vi "Q Vision_2016 Object Calcs.vi"(4 "Threshhold":i32=50, 6 "ColorMask Low/High":u8[][](array[numeric])=[[0, 100], [200, 255], [170, 230]], 7 "ColorSpace":T1, 8 "error in (no error)":errorcluster, 10 "Image in":T3) -> (0 "error out":errorcluster, 3 "Object Params out":T2 {"Deg_Up" format="%.2f"; "Deg_Rt" format="%.2f"; "Dist_ft" format="%.1f"})   [LabVIEW 2016]
uses:
  <vilib>/vision/Image Controls.llb/IMAQ Image.ctl
  Typedefs/typedef_cluster_Object Params.ctl
  Quick Vision/Typedefs/typedef_enum_ColorSpace.ctl
panel:
  out "B/W Image":i16[][](graph)
  out "Image Pixels (U32)":u32[][](array[numeric]) format="%08x"
  out "B/W Image_Object":i16[][](graph)
  # "R"
  # "G"
  # "B"
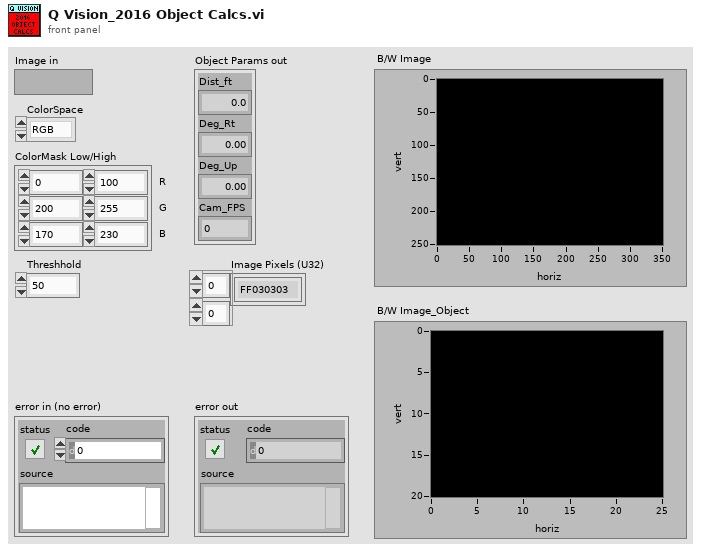
[diagram p1: front panel]
types:
  T1 = typedef "typedef_enum_ColorSpace.ctl" = enum16{"RGB", "HSL"}
  T2 = typedef "typedef_cluster_Object Params.ctl" = cluster{"Dist_ft":dbl, "Deg_Rt":dbl, "Deg_Up":dbl, "Cam_FPS":dbl}
  T3 = typedef "IMAQ Image.ctl" = refnum<image>
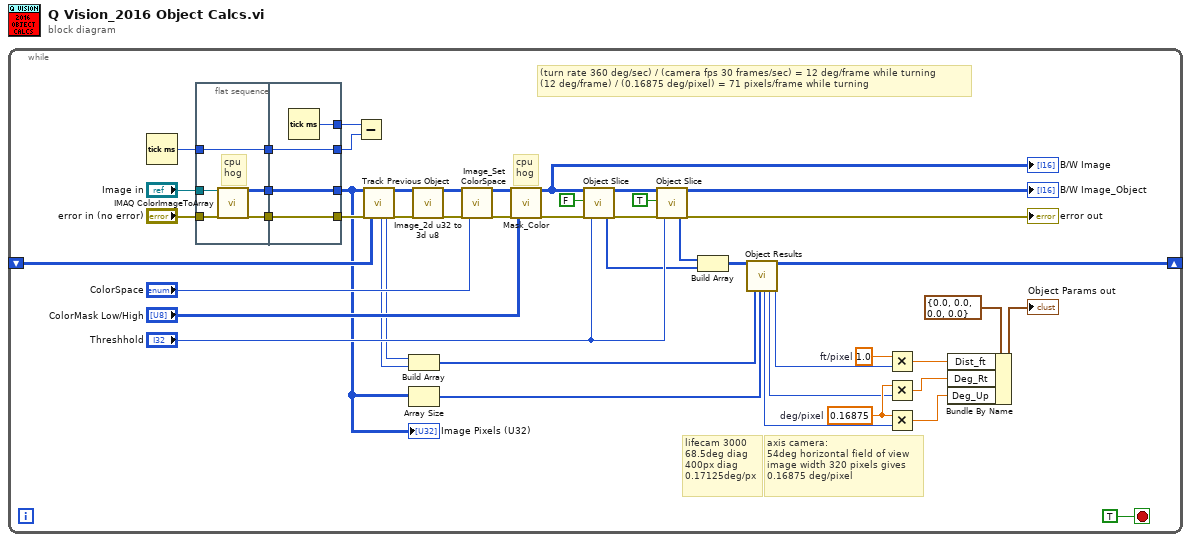
[diagram p0: block diagram]
diagram:
  n1 = while {
    shift-right: [w8] -> _
    shift-left: _ -> [w20]
    stop <- TRUE stop-if-true
    w7 = 1.0  # ft/pixel
    w28 = 0.16875  # deg/pixel
    # "lifecam 3000\n68.5deg diag\n400px diag\n0.17125deg/px"
    # "(turn rate 360 deg/sec) / (camera fps 30 frames/sec) = 12 deg/frame while turning\n(12 deg/frame) / (0.16875 deg/pixel) = 71 pixels/frame while turning"
    # "axis camera:\n54deg horizontal field of view\nimage width 320 pixels gives\n0.16875 deg/pixel"
    # "cpu\nhog"
    n2 = Tick Count (ms)() -> (millisecond timer value=w36:u32)
    n3 = flat-sequence {
      tunnel: [w52] -> w46
      tunnel: [w50] -> w45
      tunnel: [w51] -> w44
      tunnel: w36 -> [w50]
      tunnel: "Image in" -> [w49]
      tunnel: "error in (no error)" -> [w48]
      tunnel: [w54] -> w19
      tunnel: [w55] -> w30
      tunnel: [w56] -> w17
      tunnel: w46 -> [w56]
      tunnel: w45 -> [w55]
      tunnel: w44 -> [w54]
      tunnel: [w53] -> w31
      frame #0 {
        # "cpu\nhog"
        n4 = call "IMAQ ColorImageToArray"("Image"=w49, "error in (no error)"=w48) -> ("Image Pixels (U32)"=w52:u32[][], "error out"=w51:errorcluster)  [unwired: 2 in, 1 out]
      }
      frame #1 {
        n5 = Tick Count (ms)() -> (millisecond timer value=w53:u32)
      }
    }
    n6 = Subtract(x=w31, y=w30) -> ()  [unwired: 1 out]
    n7 = call "Track Previous Object.vi"("Image_2d_u32 in"=w17, "error in (no error)"=w19, "Prev. Object Start/Stop/Sum"=w20) -> ("Col Offset"=w14:i32, "Row Offset"=w15:i32, "Image_2d_u32 out"=w21:u32[][], "error out"=w18:errorcluster)  [unwired: 13 in]
    n8 = Build Array(w15, w14) -> (w2:i32[])
    n9 = Array Size(array=w17) -> (size(s)=w3:i32[])
    n10 = call "Image_2d u32 to 3d u8.vi"("Image_2d_u32"=w21, "error in (no error)"=w18) -> ("Image_3d_u8"=w42:u8[][][], "error out"=w40:errorcluster)  [unwired: 16 in]
    n11 = call "Image_Set ColorSpace.vi"("Image_3d"=w42, "error in (no error)"=w40, "ColorSpace"="ColorSpace") -> ("Image_3d_ColorSpace"=w41:u8[][][], "error out"=w43:errorcluster)  [unwired: 14 in, 1 out]
    n12 = call "Mask_Color.vi"("Image_3d"=w41, "error in (no error)"=w43, "ColorMask Low/High"="ColorMask Low/High") -> ("Image_2d"=w27:i16[][], "error out"=w39:errorcluster)  [unwired: 14 in, 1 out]
    "B/W Image" <- w27
    n13 = call "Object Slice.vi"("Image_2d"=w27, "Slice Rows(T)/Cols(F)"=FALSE, "error in (no error)"=w39, "Threshhold"="Threshhold") -> ("Object Start/Stop/Sum"=w12:i32[], "Image_2d_Slice"=w37:i16[][], "error out"=w24:errorcluster)  [unwired: 13 in]
    n14 = call "Object Slice.vi"("Image_2d"=w37, "Slice Rows(T)/Cols(F)"=TRUE, "error in (no error)"=w24, "Threshhold"="Threshhold") -> ("Object Start/Stop/Sum"=w13:i32[], "Image_2d_Slice"=→"B/W Image_Object":i16[][], "error out"=→"error out":errorcluster)  [unwired: 13 in]
    n15 = Build Array(w13, w12) -> (w9:i32[][])
    n16 = call "Object Results.vi"("Object Start/Stop/Sum in"=w9, "Offset rows,cols"=w2, "Image rows,cols"=w3) -> ("Pixels Up"=w4:i32, "Pixels Rt"=w5:i32, "Object Start/Stop/Sum out"=w8:i32[][], "Pixel Sum"=w6:i32)  [unwired: 13 in]
    n17 = Multiply(x=w7, y=w6) -> (x*y=w10:dbl)
    n18 = Multiply(x=w28, y=w5) -> (x*y=w11:dbl)
    n19 = Multiply(x=w28, y=w4) -> (x*y=w29:dbl)
    n20 = Bundle By Name(cluster=T2 {"Dist_ft"=0.0, "Deg_Rt"=0.0, "Deg_Up"=0.0, "Cam_FPS"=0.0} ("Object Params out"), "Dist_ft"=w10, "Deg_Rt"=w11, "Deg_Up"=w29) -> (→"Object Params out":T2)
    "Image Pixels (U32)" <- w17
  }
